vi "Batch Configure VIs for NI Drivers.vi"() -> ()   [LabVIEW 2025]
doc: "Instrument Driver Compliance Tool\n\nDescription:\nThe <b>Instrument Driver Compliance Tool</b> provides automated support for adjusting VI properties to meet the guidelines specified by NI in the Instrument Driver Development Tools and Resources. It ensures consistency across all driver VIs and reduces manual configuration effort.\n\nKey Rules Enforced:\n\n<b>Protection</b>: Unlocked — Users must have access to the source code for customization and extension.\n\n<b>Window Appearance</b>: Default — Guarantees consistent appearance with standard LabVIEW VIs.\n\n<b>Execution</b>:\n\nAllow Debugging: Enabled — Facilitates troubleshooting of cables, addresses, and configuration.\n\nReentrant Execution: Disabled — Avoids unnecessary memory overhead and simplifies debugging.\n\nPreferred Execution System: Same as Caller — Ensures flexibility according to application needs.\n\nAutomatic Error Handling: Disabled — Error management should be handled explicitly via error clusters.\n\nRun when Opened: Disabled — Execution should remain under user control.\n\nSuspend when Called: Disabled — Instrument Driver VIs must not suspend when invoked.\n\nUsage:\nRun this tool on VIs within an instrument driver project to validate or apply the recommended property settings automatically.\n\nBenefits:\n\nGuarantees NI-compliant driver development.\n\nSaves time by standardizing VI property settings.\n\nImproves maintainability and debugging capabilities."
panel:
  in  "Disconnect VIs From Library?":bool
  in  "Folder VIs Path":path
  # "By default, this feature is disabled. To enable it, you must modify the code in the Diagram Disable Structure."
  # "YES"
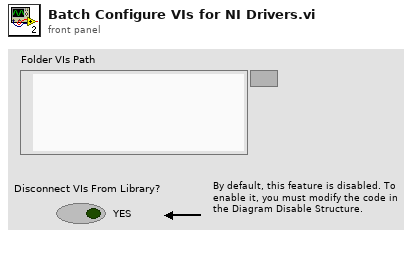
[diagram p1: front panel]
types:
  T1 = enum32{"Invalid", "Default", "Floating", "Floating/Auto-Hide", "Modal"}
  T2 = enum32{"invalid execution system", "user interface", "standard", "instrument i/o", "data acquisition", "other 1", "other 2", "same as caller"}
  T3 = enum32{"invalid lock state", "Not Locked", "Locked (No Password)", "Password-protected"}
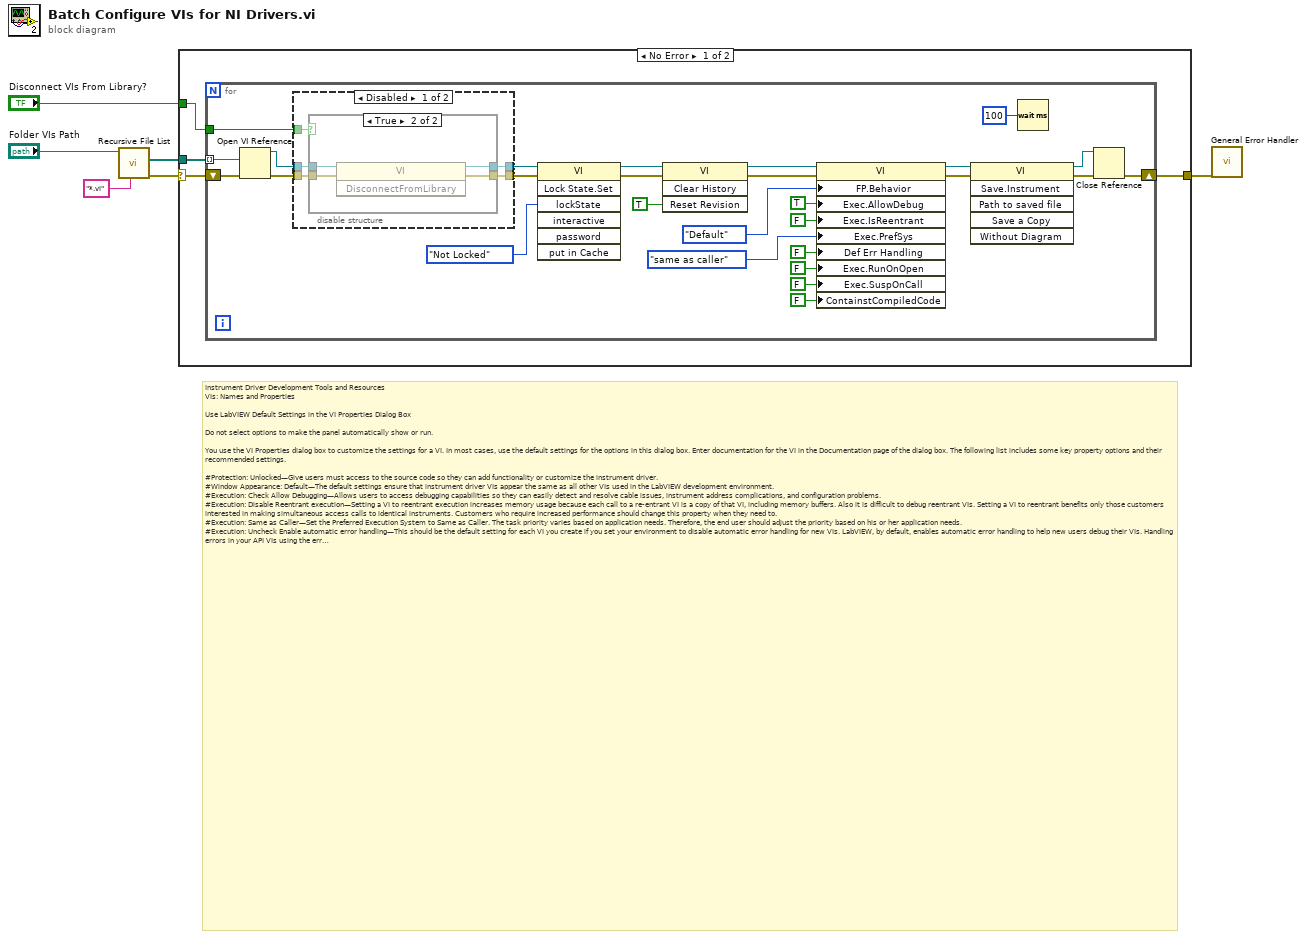
[diagram p0: block diagram]
diagram:
  # "Instrument Driver Development Tools and Resources \nVIs: Names and Properties\n \nUse LabVIEW Default Settings in the VI Properties Dialog Box\n\nDo not select options to make the panel automatically show or run.\n\nYou use the VI Properties dialog box to customize the settings for a VI. In most cases, use the default settings for the options in this dialog box. Enter documentation for the VI in the Documentation page of the dialog box. The following list includes some key property options and their recommended settings.\n\n#Protection: Unlocked—Give users must access to the source code so they can add functionality or customize the instrument driver.\n#Window Appearance: Default—The default settings ensure that instrument driver VIs appear the same as all other VIs used in the LabVIEW development environment.\n#Execution: Check Allow Debugging—Allows users to access debugging capabilities so they can easily detect and resolve cable issues, instrument address complications, and configuration problems.\n#Execution: Disable Reentrant execution—Setting a VI to reentrant execution increases memory usage because each call to a re-entrant VI is a copy of that VI, including memory buffers. Also it is difficult to debug reentrant VIs. Setting a VI to reentrant benefits only those customers interested in making simultaneous access calls to identical instruments. Customers who require increased performance should change this property when they need to.\n#Execution: Same as Caller—Set the Preferred Execution System to Same as Caller. The task priority varies based on application needs. Therefore, the end user should adjust the priority based on his or her application needs.\n#Execution: Uncheck Enable automatic error handling—This should be the default setting for each VI you create if you set your environment to disable automatic error handling for new VIs. LabVIEW, by default, enables automatic error handling to help new users debug their VIs. Handling errors in your API VIs using the error in and error out cluster parameters ensures errors are properly reported to users.\n#Execution: Uncheck Run when Opened—When used interactively, users should control when the VI runs.\n#Execution: Uncheck Suspend when Called—Instrument Driver VIs never should be suspended when called.\n\nIf you Use LabVIEW Revision History, Reset the History When Releasing Version 1.0 of the Driver\n\nRecommended\nBefore releasing version 1.0 of an instrument driver, clear the revision history of each VI. This facilitates version tracking each time someone updates the driver. To clear the revision history, choose VI Revision History from the Tools menu and click on the Reset button. Choose Yes to reset the revision number. Then close the revision history window and save the VI. Consider using the Invoke Node and the Clear History method to reset the revision history for a collection of VIs. Refer to Programmatically Controlling VIs in the LabVIEW Help for more information about configuring VIs programmatically.\n\n\nSource: https://www.ni.com/en/support/downloads/instrument-drivers/tools-resources/instrument-driver-guidelines/vis-names-and-properties.html"
  n1 = call <vilib>:"Recursive File List.vi"("pattern"="*.vi", "Folder Path"="Folder VIs Path") -> ("error out"=w1:errorcluster, "All Files in Dir"=w5:path[])  [unwired: 5 in, 3 out]
  n2 = case shown="No Error" w1 {
    selector: w1 -> [w7 w51]
    tunnel: w5 -> [w10 _]
    tunnel: [w9 w51] -> w4
    tunnel: "Disconnect VIs From Library?" -> [w8 _]
    frame No Error {
      n3 = for {
        tunnel: w10 -> [w37] mode=indexing
        shift-right: [w35] -> w9
        shift-left: w7 -> [w36]
        tunnel: w8 -> [w17]
        n4 = Open VI Reference(vi path=w37, error in (no error)=w36) -> (vi reference=w20:refnum<vi>, error out=w21:errorcluster)  [unwired: 4 in]
        n5 = disable-structure shown="Disabled" {
          disable-tunnel: w21 -> [w42 w50]
          disable-tunnel: w20 -> [w41 w49]
          disable-tunnel: [w40 w49] -> w19
          disable-tunnel: [w39 w50] -> w18
          disable-tunnel: w17 -> [w38 _]
          frame Disabled {
            n6 = case shown="True" w38 {
              tunnel: w42 -> [w44 w48]
              tunnel: w41 -> [w43 w47]
              tunnel: [w43 w46] -> w40
              tunnel: [w44 w45] -> w39
              frame False {
              }
              frame True {
                n7 = invoke class="VI" method="DisconnectFromLibrary"(reference=w47, error in=w48) -> (reference out=w46:refnum<vi>, error out=w45:errorcluster)  [unwired: 1 in, 1 out]
              }
            }
          }
          frame Enabled {
          }
        }
        n8 = invoke class="VI" method="Lock State.Set"(reference=w19, error in=w18, "lockState"=T3."Not Locked" ("Lock State")) -> (reference out=w12:refnum<vi>, error out=w14:errorcluster)  [unwired: 4 in, 5 out]
        n9 = invoke class="VI" method="Clear History"(reference=w12, error in=w14, "Reset Revision"=TRUE) -> (reference out=w11:refnum<vi>, error out=w13:errorcluster)  [unwired: 1 in, 2 out]
        n10 = property class="VI"(reference=w11, error in=w13, "FP.Behavior"=T1."Default" ("Front Panel Window:Behavior"), "Exec.AllowDebug"=TRUE ("Execution:Allow Debugging"), "Exec.IsReentrant"=FALSE ("Execution:Is Reentrant"), "Exec.PrefSys"=T2."same as caller" ("Execution:Preferred Exec System"), "Def Err Handling"=FALSE ("Automatic Error Handling"), "Exec.RunOnOpen"=FALSE ("Execution:Is Reentrant"), "Exec.SuspOnCall"=FALSE ("Execution:Suspend On Call"), "ContainstCompiledCode"=FALSE ("Contains Compiled Code")) -> (reference out=w23:refnum<vi>, error out=w22:errorcluster)
        n11 = invoke class="VI" method="Save.Instrument"(reference=w23, error in=w22) -> (reference out=w33:refnum<vi>, error out=w34:errorcluster)  [unwired: 4 in, 4 out]
        n12 = Wait (ms)(milliseconds to wait=u32 100) -> ()  [unwired: 1 out]
        n13 = Close Reference(reference=w33, error in (no error)=w34) -> (error out=w35:errorcluster)
      }
    }
    frame Error {
    }
  }
  n14 = call <vilib>:"General Error Handler.vi"("error in (no error)"=w4) -> ()  [unwired: 10 in, 5 out]
